vi "ClimberControlManager.vi"(0 "ClimbDriveDevRef":T20={"DeviceStatus"={"status"=FALSE, "code"=0, "source"=""}, "Type"=enum."PWM", "PWM"={"PWM Channel"=enum."Invalid", "DeadBand"={"Name"="", "maxPositivePwm"=0, "minPositivePwm"=0, "centerPwm"=0, "maxNegativePwm"=0, "minNegativePwm"=0, "angularRange"=0}}, "CAN"={"Device Number"=0, "SetOutput VI Ref"=variant(refnum<vi> refnum), "GetOutput VI Ref"=variant(refnum<vi> refnum), "Enable VI Ref"=variant(refnum<vi> refnum), "Disable VI Ref"=variant(refnum<vi> refnum), "Data"=variant}, "Invert"=FALSE, "DIO PWM"={"PWM \"Enable\" Channel"=enum."Invalid", "DIOChannel"=enum."Invalid", "PWM Rate"=0.0}}, 1 "FrontClimbDevRef":T20={"DeviceStatus"={"status"=FALSE, "code"=0, "source"=""}, "Type"=enum."PWM", "PWM"={"PWM Channel"=enum."Invalid", "DeadBand"={"Name"="", "maxPositivePwm"=0, "minPositivePwm"=0, "centerPwm"=0, "maxNegativePwm"=0, "minNegativePwm"=0, "angularRange"=0}}, "CAN"={"Device Number"=0, "SetOutput VI Ref"=variant(refnum<vi> refnum), "GetOutput VI Ref"=variant(refnum<vi> refnum), "Enable VI Ref"=variant(refnum<vi> refnum), "Disable VI Ref"=variant(refnum<vi> refnum), "Data"=variant}, "Invert"=FALSE, "DIO PWM"={"PWM \"Enable\" Channel"=enum."Invalid", "DIOChannel"=enum."Invalid", "PWM Rate"=0.0}}, 2 "RearClimbDevRef":T20={"DeviceStatus"={"status"=FALSE, "code"=0, "source"=""}, "Type"=enum."PWM", "PWM"={"PWM Channel"=enum."Invalid", "DeadBand"={"Name"="", "maxPositivePwm"=0, "minPositivePwm"=0, "centerPwm"=0, "maxNegativePwm"=0, "minNegativePwm"=0, "angularRange"=0}}, "CAN"={"Device Number"=0, "SetOutput VI Ref"=variant(refnum<vi> refnum), "GetOutput VI Ref"=variant(refnum<vi> refnum), "Enable VI Ref"=variant(refnum<vi> refnum), "Disable VI Ref"=variant(refnum<vi> refnum), "Data"=variant}, "Invert"=FALSE, "DIO PWM"={"PWM \"Enable\" Channel"=enum."Invalid", "DIOChannel"=enum."Invalid", "PWM Rate"=0.0}}, 3 "ClimbDriveManualControl":dbl, 4 "FrontClimbManualControl":dbl, 5 "RearClimbManualControl":dbl, 6 "Climb Positions":T16, 7 "FrontClimberPosition":T18, 8 "Climber Home State":T19, 9 "RearClimberPosition":T18, 10 "RobotConfig":T2={"Motors"={"DriveRightPrimary"={"CAN Address"=1, "Invert"=FALSE, "InvertSensor"=FALSE, "Unit Conversion Factor"=0.0, "Brake Mode"=enum."Override to Brake", "Reverse Limt Switch Mode"=enum."Normally Closed", "Forward Limt Swith Mode"=enum."Normally Closed", "PWM Channel"=enum."Invalid", "Motor Controller Type"=enum."Talon SRX", "Peak Current (A)"=0, "Continuos Current (A)"=0, "Peak Duration (ms)"=0, "Current Limit Enable"=FALSE}, "DriveRightSecondary"={"CAN Address"=2, "Invert"=FALSE, "InvertSensor"=FALSE, "Unit Conversion Factor"=0.0, "Brake Mode"=enum."Override to Brake", "Reverse Limt Switch Mode"=enum."Normally Closed", "Forward Limt Swith Mode"=enum."Normally Closed", "PWM Channel"=enum."Invalid", "Motor Controller Type"=enum."Talon SRX", "Peak Current (A)"=0, "Continuos Current (A)"=0, "Peak Duration (ms)"=0, "Current Limit Enable"=FALSE}, "DriveLeftPrimary"={"CAN Address"=3, "Invert"=FALSE, "InvertSensor"=FALSE, "Unit Conversion Factor"=0.0, "Brake Mode"=enum."Override to Brake", "Reverse Limt Switch Mode"=enum."Normally Closed", "Forward Limt Swith Mode"=enum."Normally Closed", "PWM Channel"=enum."Invalid", "Motor Controller Type"=enum."Talon SRX", "Peak Current (A)"=0, "Continuos Current (A)"=0, "Peak Duration (ms)"=0, "Current Limit Enable"=FALSE}, "DriveLeftSecondary"={"CAN Address"=4, "Invert"=FALSE, "InvertSensor"=FALSE, "Unit Conversion Factor"=0.0, "Brake Mode"=enum."Override to Brake", "Reverse Limt Switch Mode"=enum."Normally Closed", "Forward Limt Swith Mode"=enum."Normally Closed", "PWM Channel"=enum."Invalid", "Motor Controller Type"=enum."Talon SRX", "Peak Current (A)"=0, "Continuos Current (A)"=0, "Peak Duration (ms)"=0, "Current Limit Enable"=FALSE}, "RearClimb"={"CAN Address"=8, "Invert"=FALSE, "InvertSensor"=FALSE, "Unit Conversion Factor"=0.0, "Brake Mode"=enum."Override to Brake", "Reverse Limt Switch Mode"=enum."Normally Closed", "Forward Limt Swith Mode"=enum."Normally Closed", "PWM Channel"=enum."Invalid", "Motor Controller Type"=enum."Talon SRX", "Peak Current (A)"=0, "Continuos Current (A)"=0, "Peak Duration (ms)"=0, "Current Limit Enable"=FALSE}, "Front Climb"={"CAN Address"=7, "Invert"=FALSE, "InvertSensor"=FALSE, "Unit Conversion Factor"=0.0, "Brake Mode"=enum."Override to Brake", "Reverse Limt Switch Mode"=enum."Normally Closed", "Forward Limt Swith Mode"=enum."Normally Closed", "PWM Channel"=enum."Invalid", "Motor Controller Type"=enum."Talon SRX", "Peak Current (A)"=0, "Continuos Current (A)"=0, "Peak Duration (ms)"=0, "Current Limit Enable"=FALSE}, "Climb Drive"={"CAN Address"=5, "Invert"=FALSE, "InvertSensor"=FALSE, "Unit Conversion Factor"=0.0, "Brake Mode"=enum."Override to Brake", "Reverse Limt Switch Mode"=enum."Normally Closed", "Forward Limt Swith Mode"=enum."Normally Closed", "PWM Channel"=enum."Invalid", "Motor Controller Type"=enum."Talon SRX", "Peak Current (A)"=0, "Continuos Current (A)"=0, "Peak Duration (ms)"=0, "Current Limit Enable"=FALSE}, "Shoulder1"={"CAN Address"=6, "Invert"=FALSE, "InvertSensor"=FALSE, "Unit Conversion Factor"=0.0, "Brake Mode"=enum."Override to Brake", "Reverse Limt Switch Mode"=enum."Normally Closed", "Forward Limt Swith Mode"=enum."Normally Closed", "PWM Channel"=enum."Invalid", "Motor Controller Type"=enum."Talon SRX", "Peak Current (A)"=0, "Continuos Current (A)"=0, "Peak Duration (ms)"=0, "Current Limit Enable"=FALSE}, "Shoulder2"={"CAN Address"=9, "Invert"=FALSE, "InvertSensor"=FALSE, "Unit Conversion Factor"=0.0, "Brake Mode"=enum."Override to Brake", "Reverse Limt Switch Mode"=enum."Normally Closed", "Forward Limt Swith Mode"=enum."Normally Closed", "PWM Channel"=enum."Invalid", "Motor Controller Type"=enum."Talon SRX", "Peak Current (A)"=0, "Continuos Current (A)"=0, "Peak Duration (ms)"=0, "Current Limit Enable"=FALSE}, "Wrist"={"CAN Address"=10, "Invert"=FALSE, "InvertSensor"=FALSE, "Unit Conversion Factor"=0.0, "Brake Mode"=enum."Override to Brake", "Reverse Limt Switch Mode"=enum."Disabled", "Forward Limt Swith Mode"=enum."Disabled", "PWM Channel"=enum."Invalid", "Motor Controller Type"=enum."Talon SRX", "Peak Current (A)"=0, "Continuos Current (A)"=0, "Peak Duration (ms)"=0, "Current Limit Enable"=FALSE}, "Extension"={"CAN Address"=11, "Invert"=FALSE, "InvertSensor"=FALSE, "Unit Conversion Factor"=0.0, "Brake Mode"=enum."Override to Brake", "Reverse Limt Switch Mode"=enum."Disabled", "Forward Limt Swith Mode"=enum."Disabled", "PWM Channel"=enum."Invalid", "Motor Controller Type"=enum."Talon SRX", "Peak Current (A)"=0, "Continuos Current (A)"=0, "Peak Duration (ms)"=0, "Current Limit Enable"=FALSE}, "CargoIntake"={"CAN Address"=11, "Invert"=FALSE, "InvertSensor"=FALSE, "Unit Conversion Factor"=0.0, "Brake Mode"=enum."Override to Brake", "Reverse Limt Switch Mode"=enum."Disabled", "Forward Limt Swith Mode"=enum."Disabled", "PWM Channel"=enum."Invalid", "Motor Controller Type"=enum."Talon SRX", "Peak Current (A)"=0, "Continuos Current (A)"=0, "Peak Duration (ms)"=0, "Current Limit Enable"=FALSE}, "Intake2"={"CAN Address"=11, "Invert"=FALSE, "InvertSensor"=FALSE, "Unit Conversion Factor"=0.0, "Brake Mode"=enum."Override to Brake", "Reverse Limt Switch Mode"=enum."Disabled", "Forward Limt Swith Mode"=enum."Disabled", "PWM Channel"=enum."Invalid", "Motor Controller Type"=enum."Talon SRX", "Peak Current (A)"=0, "Continuos Current (A)"=0, "Peak Duration (ms)"=0, "Current Limit Enable"=FALSE}}, "Sensors"={"IMU"={"Yaw Axis"=enum."Z", "SPI Bus"=enum."SPI MXP", "AHRS Algorithm"=enum."Complementary", "Calibration Time (s)"=3.0, "Calibrate On Open"=TRUE}}, "PID"={"FrontClimb"={"P"=0.0, "I"=0.0, "D"=0.0, "F"=0.0, "IZone"=0.0}, "RearClimb"={"P"=0.0, "I"=0.0, "D"=0.0, "F"=0.0, "IZone"=0.0}, "ArmShoulder"={"P"=0.0, "I"=0.0, "D"=0.0, "F"=0.0, "IZone"=0.0}, "ArmExtend"={"P"=0.0, "I"=0.0, "D"=0.0, "F"=0.0, "IZone"=0.0}, "ArmWrist"={"P"=0.0, "I"=0.0, "D"=0.0, "F"=0.0, "IZone"=0.0}}, "Solenoids"={" Shifter"={"SolenoidChannel"=enum."Solenoid 3", "Invert"=FALSE}, "Hatch Grip"={"SolenoidChannel"=enum."Solenoid 0", "Invert"=FALSE}, "Hatch Extend"={"SolenoidChannel"=enum."Solenoid 0", "Invert"=FALSE}, "Manipulator Slide"={"SolenoidChannel"=enum."Solenoid 0", "Invert"=FALSE}, "Hatch Floor Intake"={"SolenoidChannel"=enum."Solenoid 0", "Invert"=FALSE}}, "Enable Compressor"=TRUE, "MotionMagic"={"FrontClimb"={"CruiseVelocity"=0, "Acceleration"=0}, "RearClimb"={"CruiseVelocity"=0, "Acceleration"=0}}, "RobotDimensions"={"Length (in)"=0.0, "Shoulder Height (in)"=0.0, "Frame Height (in)"=0.0, "Arm Center to Front of Robot (in)"=0.0, "Arm Min Extension (in)"=0.0, "Arm Max Extension (in)"=0.0}, "Arm Home Position"={"Radius (in)"=0.0, "ShoulderAngle (rad)"=0.0, "WristAngle (rad)"=0.0}, "Climb Home Position"={"Back Climb"=0.0, "Front Climb"=0.0}, "Climb Positions"={"Retract"=0.0, "Level 2"=0.0, "Level 3"=0.0}}, 11 "AutoClimbDrive":dbl, 12 "AutoClimbState":T1, 13 "AutoControlStart":bool) -> (14 "ClimbMode":T17)   [LabVIEW 2018]
uses:
  <vilib>/Rock Robotics/WPI/MotorControl/WPI_MotorControlDeviceRef.ctl
  <vilib>/Rock Robotics/WPI/MotorControl/WPI_MotorControlType.ctl
  <vilib>/Rock Robotics/SystemInterfaces/DIO/FPGA_DIOPWMChannel.ctl
  <vilib>/Rock Robotics/WPI/PWM/WPI_PWMDeadband.ctl
  <vilib>/Rock Robotics/SystemInterfaces/DIO/FPGA_DIOChannel.ctl
  TypeDefs/ClimberHomingState.ctl
  TypeDefs/ClimberPositionHeights.ctl
  TypeDefs/ClimberPositions.ctl
  TypeDefs/ClimberMode.ctl
  TypeDefs/ConfigComponents/Config_Robot.ctl
  ArgosLib/Config/ConfigComponents/TypeDefs/Config_Motor.ctl
  <vilib>/Rock Robotics/WPI/ThirdParty/Phoenix-LabVIEW/Motor Controller/Controls/CTRE_Phoenix_MotorControl_NeutralMode.ctl
  <vilib>/Rock Robotics/WPI/ThirdParty/Phoenix-LabVIEW/Motor Controller/Controls/CTRE_Phoenix_MotorControl_LimitSwitchNormal.ctl
  ArgosLib/Config/ConfigComponents/TypeDefs/Config_MotorCtrlType.ctl
  ArgosLib/Config/ConfigComponents/TypeDefs/Config_IMU.ctl
  <vilib>/Rock Robotics/SystemInterfaces/spilib/spi_bus.ctl
  ArgosLib/Config/ConfigComponents/TypeDefs/Config_PIDParams.ctl
  ArgosLib/Config/ConfigComponents/TypeDefs/Config_SingleSolenoid.ctl
  <vilib>/Rock Robotics/WPI/Solenoid/WPI_SolenoidChannel.ctl
  ArgosLib/Config/ConfigComponents/TypeDefs/Config_MotionMagicParams.ctl
  TypeDefs/ConfigComponents/Config_Dimensions.ctl
  Arm/TypeDefs/ArmCoordinate.ctl
  TypeDefs/ClimberStates.ctl
  <vilib>/Rock Robotics/WPI/ThirdParty/Phoenix-LabVIEW/Motor Controller/Controls/CTRE_Phoenix_MotorControl_ControlMode.ctl
  ArgosLib/ArgosLib.lvlib
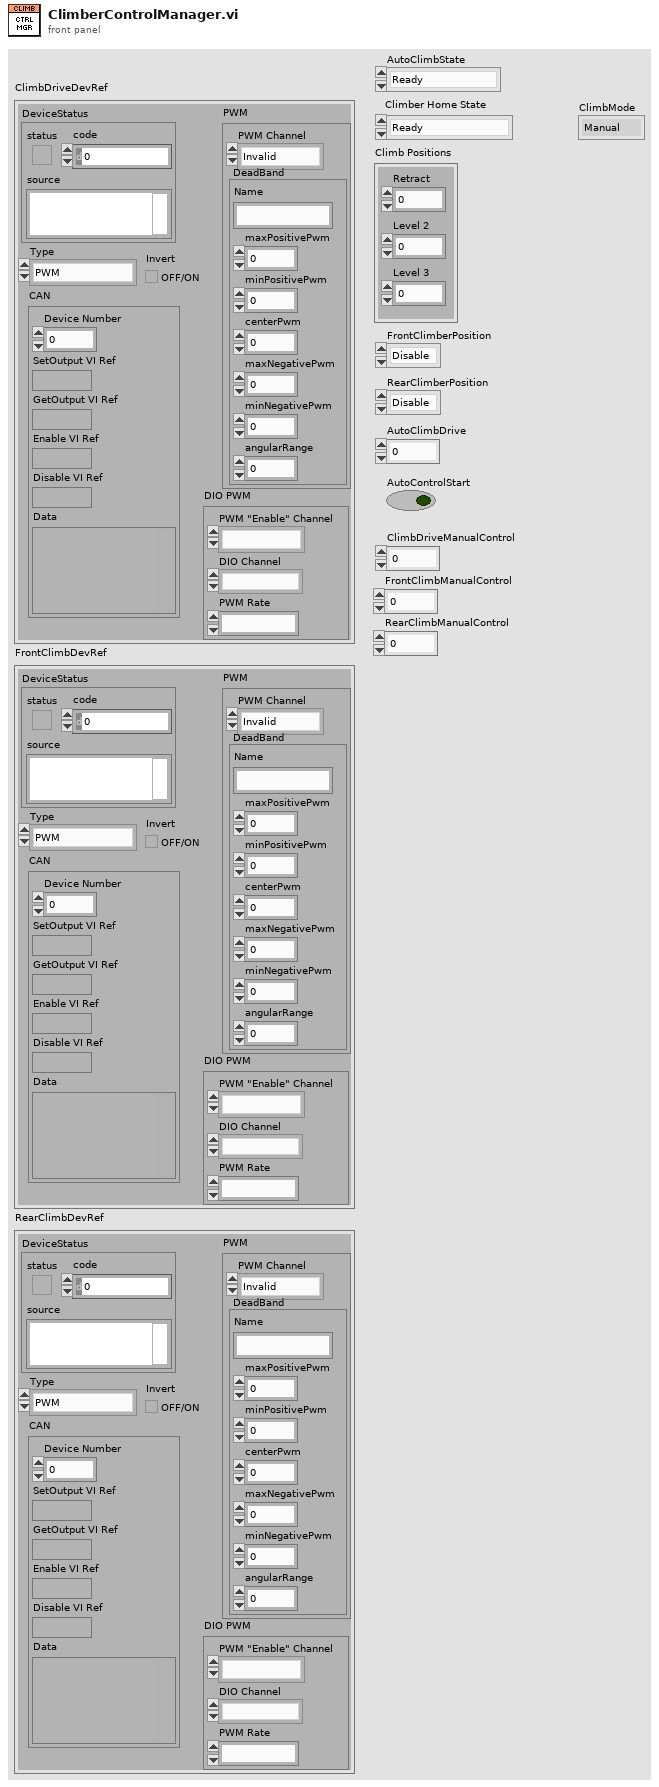
[diagram p1: front panel]
types:
  T1 = typedef "ClimberStates.ctl" = enum16{"Ready ", "Lift Bot ", "Raised Drive", "Raise Front Sticks ", "Raise Back Sticks ", "Park ", "Cancel"}
  T2 = typedef "Config_Robot.ctl" = cluster{"Motors":cluster{"DriveRightPrimary":T3, "DriveRightSecondary":T3, "DriveLeftPrimary":T3, "DriveLeftSecondary":T3, "RearClimb":T3, "Front Climb":T3, "Climb Drive":T3, "Shoulder1":T3, "Shoulder2":T3, "Wrist":T3, "Extension":T3, "CargoIntake":T3, "Intake2":T3}, "Sensors":cluster{"IMU":T8}, "PID":cluster{"FrontClimb":T10, "RearClimb":T10, "ArmShoulder":T10, "ArmExtend":T10, "ArmWrist":T10}, "Solenoids":cluster{" Shifter":T11, "Hatch Grip":T11, "Hatch Extend":T11, "Manipulator Slide":T11, "Hatch Floor Intake":T11}, "Enable Compressor":bool, "MotionMagic":cluster{"FrontClimb":T13, "RearClimb":T13}, "RobotDimensions":T14, "Arm Home Position":T15, "Climb Home Position":cluster{"Back Climb":dbl, "Front Climb":dbl}, "Climb Positions":T16}
  T3 = typedef "ArgosLib.lvlib/Config_Motor.ctl" = cluster{"CAN Address":u8, "Invert":bool, "InvertSensor":bool, "Unit Conversion Factor":dbl, "Brake Mode":T4, "Reverse Limt Switch Mode":T5, "Forward Limt Swith Mode":T5, "PWM Channel":T6, "Motor Controller Type":T7, "Peak Current (A)":i32, "Continuos Current (A)":i32, "Peak Duration (ms)":i32, "Current Limit Enable":bool}
  T4 = typedef "CTRE_Phoenix_MotorControl_NeutralMode.ctl" = enum8{"EEPROMSetting", "Override to Coast", "Override to Brake"}
  T5 = typedef "CTRE_Phoenix_MotorControl_LimitSwitchNormal.ctl" = enum16{"Normally Open", "Normally Closed", "Disabled"}
  T6 = typedef "FPGA_DIOPWMChannel.ctl" = enum8{"PWM 0", "PWM 1", "PWM 2", "PWM 3", "PWM 4", "PWM 5", "PWM 6", "PWM 7", "PWM 8", "PWM 9", "PWM MXP 0", "PWM MXP 1", "PWM MXP 2", "PWM MXP 3", "PWM MXP 4", "PWM MXP 5", "PWM MXP 6", "PWM MXP 7", "PWM MXP 8", "PWM MXP 9", "Invalid"}
  T7 = typedef "ArgosLib.lvlib/Config_MotorCtrlType.ctl" = enum16{"Disabled", "Talon SRX", "Talon SR"}
  T8 = typedef "ArgosLib.lvlib/Config_IMU.ctl" = cluster{"Yaw Axis":enum16{"X", "Y", "Z"}, "SPI Bus":T9, "AHRS Algorithm":enum16{"Complementary", "Madgwick"}, "Calibration Time (s)":dbl, "Calibrate On Open":bool}
  T9 = typedef "spi_bus.ctl" = enum16{"SPI On-Board, CS0", "SPI On-Board, CS1", "SPI On-Board, CS2", "SPI On-Board, CS3", "SPI MXP", "Invalid"}
  T10 = typedef "ArgosLib.lvlib/Config_PIDParams.ctl" = cluster{"P":dbl, "I":dbl, "D":dbl, "F":dbl, "IZone":dbl}
  T11 = typedef "ArgosLib.lvlib/Config_SingleSolenoid.ctl" = cluster{"SolenoidChannel":T12, "Invert":bool}
  T12 = typedef "WPI_SolenoidChannel.ctl" = enum8{"Solenoid 0", "Solenoid 1", "Solenoid 2", "Solenoid 3", "Solenoid 4", "Solenoid 5", "Solenoid 6", "Solenoid 7", "Invalid"}
  T13 = typedef "Config_MotionMagicParams.ctl" = cluster{"CruiseVelocity":i32, "Acceleration":i32}
  T14 = typedef "Config_Dimensions.ctl" = cluster{"Length (in)":dbl, "Shoulder Height (in)":dbl, "Frame Height (in)":dbl, "Arm Center to Front of Robot (in)":dbl, "Arm Min Extension (in)":dbl, "Arm Max Extension (in)":dbl}
  T15 = typedef "ArmCoordinate.ctl" = cluster{"Radius (in)":dbl, "ShoulderAngle (rad)":dbl, "WristAngle (rad)":dbl}
  T16 = typedef "ClimberPositionHeights.ctl" = cluster{"Retract":dbl, "Level 2":dbl, "Level 3":dbl}
  T17 = typedef "ClimberMode.ctl" = enum16{"Manual", "Auto", "Homing"}
  T18 = typedef "ClimberPositions.ctl" = enum16{"Disable", "Floor", "Level 2", "Level 3"}
  T19 = typedef "ClimberHomingState.ctl" = enum16{"Ready", "Homing In progress", "Homing Failure", "Homing Success "}
  T20 = typedef "WPI_MotorControlDeviceRef.ctl" = cluster{"DeviceStatus":errorcluster, "Type":T21, "PWM":cluster{"PWM Channel":T6, "DeadBand":T22}, "CAN":cluster{"Device Number":u8, "SetOutput VI Ref":variant, "GetOutput VI Ref":variant, "Enable VI Ref":variant, "Disable VI Ref":variant, "Data":variant}, "Invert":bool, "DIO PWM":cluster{"PWM \"Enable\" Channel":T6, "DIOChannel":T23, "PWM Rate":dbl}}
  T21 = typedef "WPI_MotorControlType.ctl" = enum16{"PWM", "CAN", "DIO PWM"}
  T22 = typedef "WPI_PWMDeadband.ctl" = cluster{"Name":string, "maxPositivePwm":i32, "minPositivePwm":i32, "centerPwm":i32, "maxNegativePwm":i32, "minNegativePwm":i32, "angularRange":u16}
  T23 = typedef "FPGA_DIOChannel.ctl" = enum8{"DIO 0", "DIO 1", "DIO 2", "DIO 3", "DIO 4", "DIO 5", "DIO 6", "DIO 7", "DIO 8", "DIO 9", "DIO MXP 0", "DIO MXP 1", "DIO MXP 2", "DIO MXP 3", "DIO MXP 4", "DIO MXP 5", "DIO MXP 6", "DIO MXP 7", "DIO MXP 8", "DIO MXP 9", "DIO MXP 10", "DIO MXP 11", "DIO MXP 12", "DIO MXP 13", "DIO MXP 14", "DIO MXP 15", "SPI Port CS1", "SPI Port CS2", "SPI Port CS3", "SPI Port MISO", "SPI Port MOSI", "Invalid"}
  T24 = typedef "CTRE_Phoenix_MotorControl_ControlMode.ctl" = u16
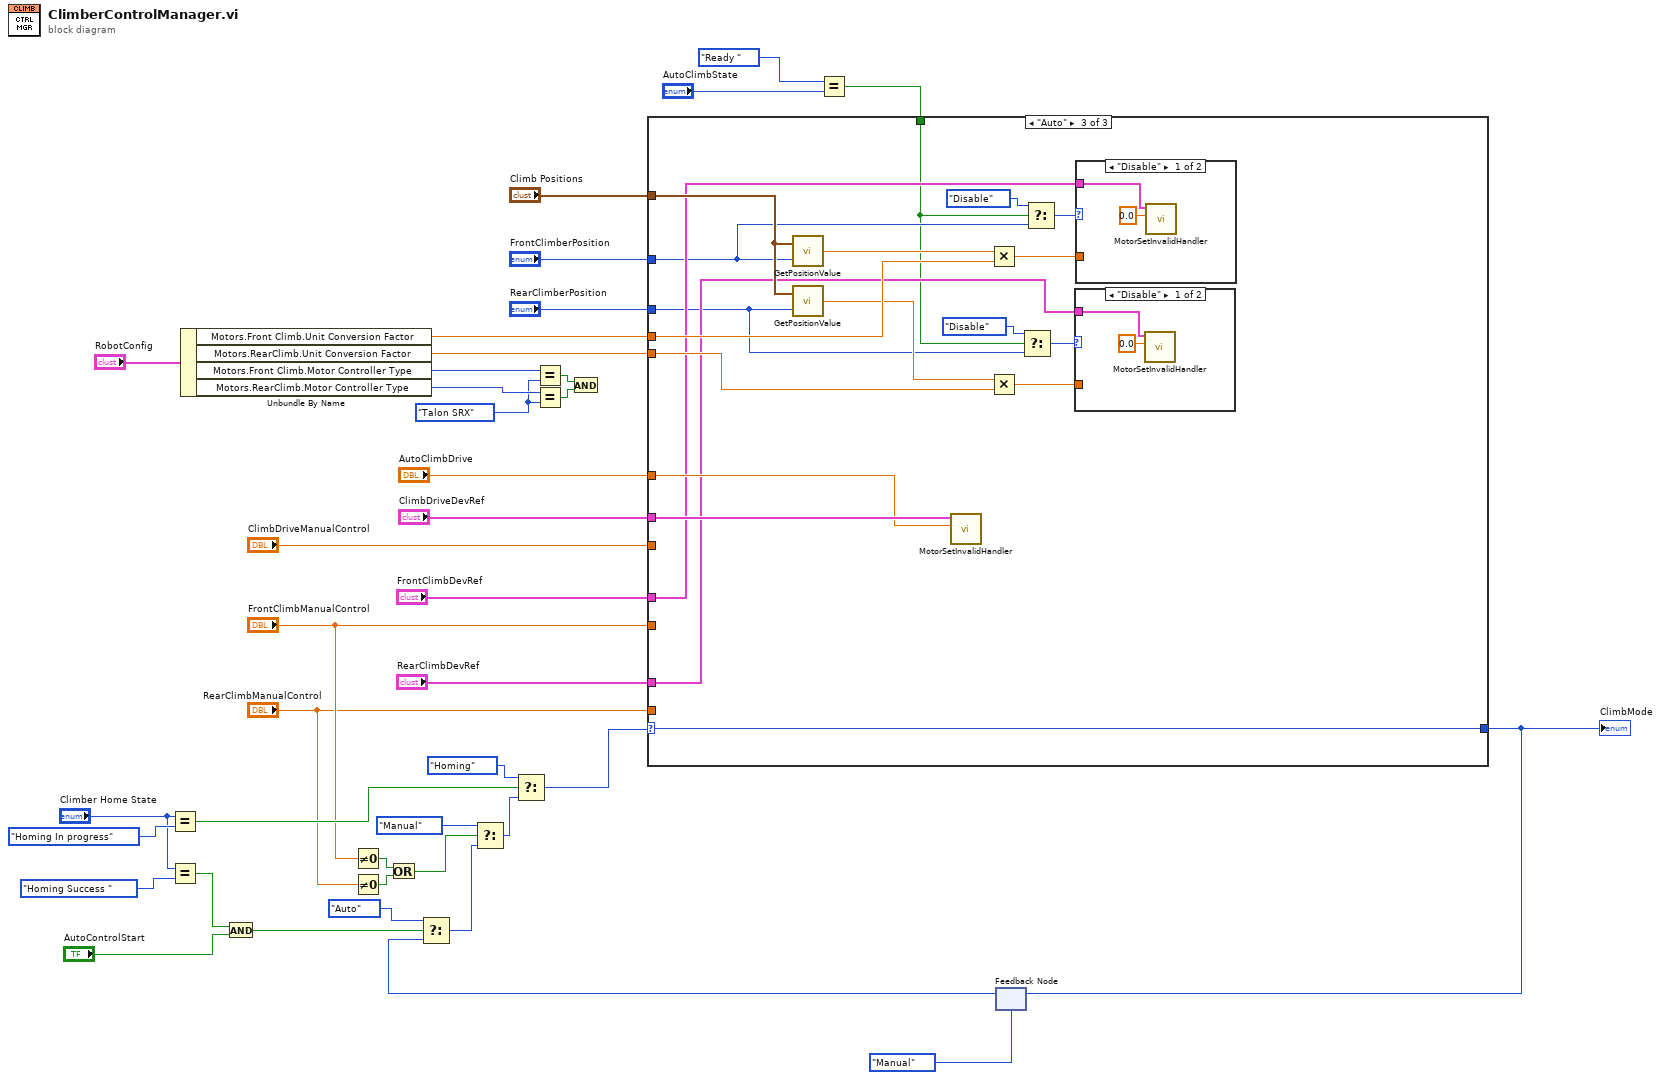
[diagram p0: block diagram]
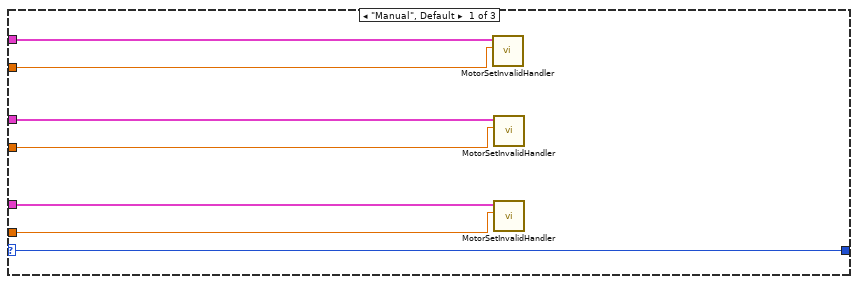
[diagram p2: hidden frame]
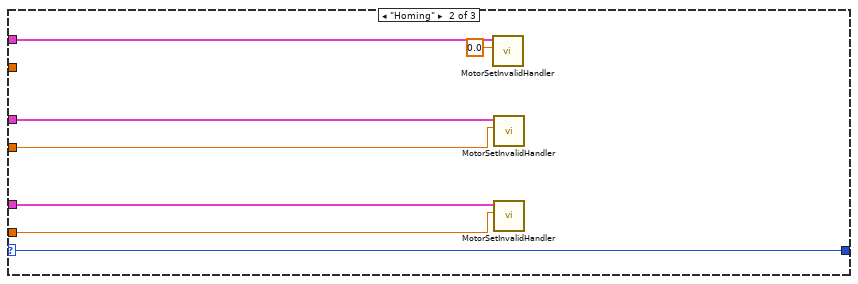
[diagram p3: hidden frame]
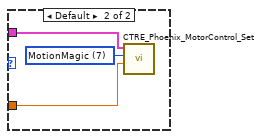
[diagram p4: hidden frame]
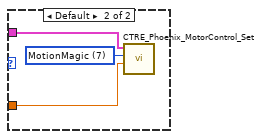
[diagram p5: hidden frame]
diagram:
  w27 = Config_MotorCtrlType."Talon SRX" ("y")
  n1 = Equal?(x="Climber Home State", y=ClimberHomingState."Homing In progress") -> (x = y?=w19:bool)
  n2 = Equal?(x="Climber Home State", y=ClimberHomingState."Homing Success ") -> (x = y?=w8:bool)
  n3 = Unbundle By Name("RobotConfig") -> ("Motors.Front Climb.Unit Conversion Factor"=w24:dbl, "Motors.RearClimb.Unit Conversion Factor"=w23:dbl, "Motors.Front Climb.Motor Controller Type"=w28:T7, "Motors.RearClimb.Motor Controller Type"=w29:T7)
  n4 = And(x=w8, y="AutoControlStart") -> (x .and. y?=w4:bool)
  n5 = Not Equal To 0?(x="FrontClimbManualControl") -> (x != 0?=w15:bool)
  n6 = Not Equal To 0?(x="RearClimbManualControl") -> (x != 0?=w14:bool)
  n7 = Or(x=w15, y=w14) -> (x .or. y?=w12:bool)
  n8 = Equal?(x=w28, y=w27) -> (x = y?=w26:bool)
  n9 = Equal?(x=w29, y=w27) -> (x = y?=w25:bool)
  n10 = And(x=w26, y=w25) -> ()  [unwired: 1 out]
  n11 = Equal?(x=ClimberStates."Ready ", y="AutoClimbState") -> (x = y?=w1:bool)
  n12 = feedback #1(ClimberMode."Manual" ("ClimbMode")) -> (w9:T17)
  n13 = Select(t=ClimberMode."Auto", s=w4, f=w9) -> (s? t:f=w10:T17)
  n14 = Select(t=ClimberMode."Manual" ("ClimbMode"), s=w12, f=w10) -> (s? t:f=w13:T17)
  n15 = Select(t=ClimberMode."Homing" ("ClimbMode"), s=w19, f=w13) -> (s? t:f=w6:T17)
  n16 = case shown="\"Auto\"" w6 {
    selector: w6 -> [w41 w49 w62]
    tunnel: "RearClimbManualControl" -> [w47 w54 _]
    tunnel: "RearClimbDevRef" -> [w46 w53 w64]
    tunnel: "FrontClimbManualControl" -> [w45 w52 _]
    tunnel: "FrontClimbDevRef" -> [w44 w51 w65]
    tunnel: "ClimbDriveManualControl" -> [w43 _ _]
    tunnel: "ClimbDriveDevRef" -> [w42 w50 w73]
    tunnel: [w41 w49 w62] -> w35
    tunnel: "AutoClimbDrive" -> [_ _ w72]
    tunnel: "FrontClimberPosition" -> [_ _ w61]
    tunnel: "RearClimberPosition" -> [_ _ w57]
    tunnel: "Climb Positions" -> [_ _ w71]
    tunnel: w24 -> [_ _ w68]
    tunnel: w23 -> [_ _ w67]
    tunnel: w1 -> [_ _ w55]
    frame "Manual", Default {
      n17 = call "MotorSetInvalidHandler.vi"("Output"=w43, "MotorControlDevRef"=w42) -> ()  [unwired: 7 in, 3 out]
      n18 = call "MotorSetInvalidHandler.vi"("Output"=w45, "MotorControlDevRef"=w44) -> ()  [unwired: 7 in, 3 out]
      n19 = call "MotorSetInvalidHandler.vi"("Output"=w47, "MotorControlDevRef"=w46) -> ()  [unwired: 7 in, 3 out]
    }
    frame "Homing" {
      n20 = call "MotorSetInvalidHandler.vi"("Output"=0.0, "MotorControlDevRef"=w50) -> ()  [unwired: 7 in, 3 out]
      n21 = call "MotorSetInvalidHandler.vi"("Output"=w52, "MotorControlDevRef"=w51) -> ()  [unwired: 7 in, 3 out]
      n22 = call "MotorSetInvalidHandler.vi"("Output"=w54, "MotorControlDevRef"=w53) -> ()  [unwired: 7 in, 3 out]
    }
    frame "Auto" {
      n23 = call "GetPositionValue.vi"("DesiredPosition"=w61, "Climb Heights"=w71) -> ("PositionHeight"=w69:dbl)
      n24 = call "GetPositionValue.vi"("DesiredPosition"=w57, "Climb Heights"=w71) -> ("PositionHeight"=w66:dbl)
      n25 = call "MotorSetInvalidHandler.vi"("Output"=w72, "MotorControlDevRef"=w73) -> ()  [unwired: 7 in, 3 out]
      n26 = Multiply(x=w69, y=w68) -> (x*y=w70:dbl)
      n27 = Multiply(x=w66, y=w67) -> (x*y=w63:dbl)
      n28 = Select(t=ClimberPositions."Disable", s=w55, f=w57) -> (s? t:f=w56:T18)
      n29 = Select(t=ClimberPositions."Disable", s=w55, f=w61) -> (s? t:f=w60:T18)
      n30 = case shown="\"Disable\"" w56 {
        tunnel: w63 -> [_ w76]
        tunnel: w64 -> [w75 w77]
        frame "Disable" {
          n31 = call "MotorSetInvalidHandler.vi"("Output"=0.0, "MotorControlDevRef"=w75) -> ()  [unwired: 7 in, 3 out]
        }
        frame Default {
          w78 = T24 7 items=["PercentOutput"=0, "Position"=1, "Velocity"=2, "Current"=3, "Follower"=5, "MotionProfile"=6, "MotionMagic"=7, "MotionProfileArc"=10, "Disabled"=15] ("Control Mode")
          n32 = call <vilib>:"CTRE_Phoenix_MotorControl_Set.vi"("Output"=w76, "Control Mode"=w78, "PhoenixMotorControlDevRef"=w77) -> ()  [unwired: 7 in, 2 out]
        }
      }
      n33 = case shown="\"Disable\"" w60 {
        tunnel: w70 -> [_ w81]
        tunnel: w65 -> [w80 w82]
        frame "Disable" {
          n34 = call "MotorSetInvalidHandler.vi"("Output"=0.0, "MotorControlDevRef"=w80) -> ()  [unwired: 7 in, 3 out]
        }
        frame Default {
          w83 = T24 7 items=["PercentOutput"=0, "Position"=1, "Velocity"=2, "Current"=3, "Follower"=5, "MotionProfile"=6, "MotionMagic"=7, "MotionProfileArc"=10, "Disabled"=15] ("Control Mode")
          n35 = call <vilib>:"CTRE_Phoenix_MotorControl_Set.vi"("Output"=w81, "Control Mode"=w83, "PhoenixMotorControlDevRef"=w82) -> ()  [unwired: 7 in, 2 out]
        }
      }
    }
  }
  "ClimbMode" <- w35
  n36 = feedback-in #1(w35) -> ()
